vi "SubVI_Overlay Line(Offset) #.vi"(5 "ROI Descriptor":T2 {"Contours"."Type" items=["No Selection", "Point", "Line", "Rectangle", "Oval", "Polygon", "Freehand Region", "Annulus", "Unused2", "Unused3", "Broken Line", "Freehand Line", "Rotated Rectangle"]}, 7 "Perpendicular Line":T1, 9 "Fit Line":T1) -> (6 "Perpendicular Line(Offset)":T1, 8 "Fit Line(Offset)":T1)   [LabVIEW 2013]
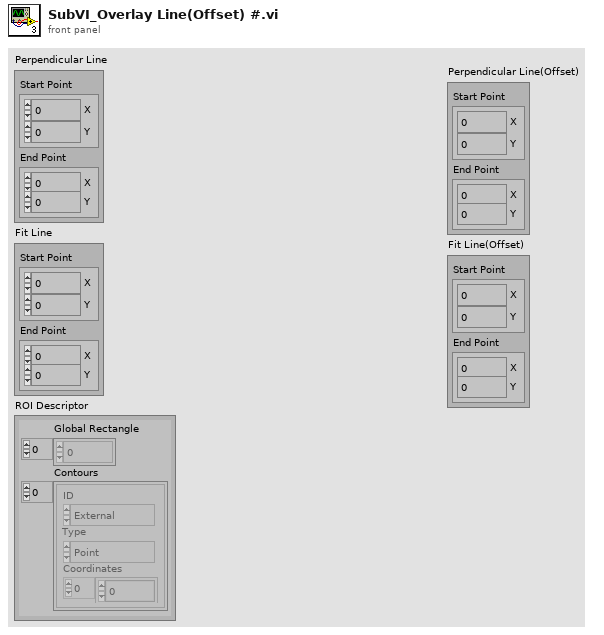
[diagram p1: front panel]
types:
  T1 = cluster{"Start Point":cluster{"X":i32, "Y":i32}, "End Point":cluster{"X":i32, "Y":i32}}
  T2 = typedef "ROI Descriptor" = cluster{"Global Rectangle":i32[], "Contours":cluster{"ID":enum32{"External", "Internal"}, "Type":u32, "Coordinates":i32[]}[]}
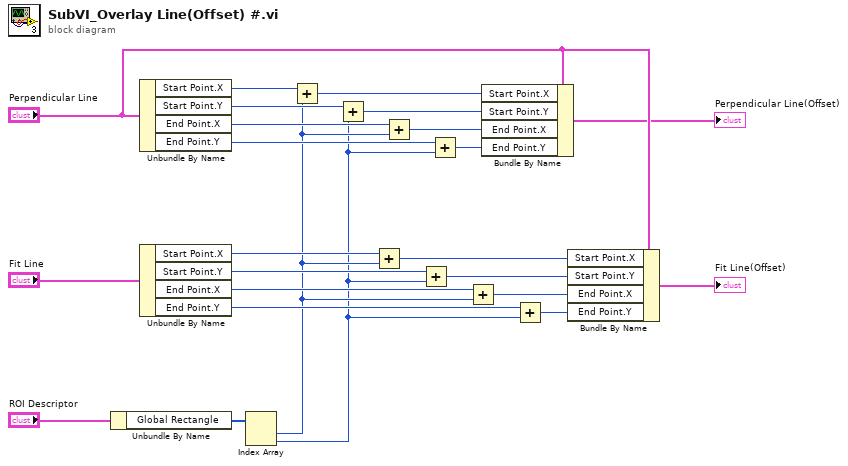
[diagram p0: block diagram]
diagram:
  n1 = Unbundle By Name("ROI Descriptor") -> ("Global Rectangle"=w22:i32[])
  n2 = Unbundle By Name("Perpendicular Line") -> ("Start Point.X"=w21:i32, "Start Point.Y"=w19:i32, "End Point.X"=w12:i32, "End Point.Y"=w11:i32)
  n3 = Unbundle By Name("Fit Line") -> ("Start Point.X"=w20:i32, "Start Point.Y"=w18:i32, "End Point.X"=w8:i32, "End Point.Y"=w7:i32)
  n4 = Index Array(array=w22) -> (element #1=w6:i32, element #2=w5:i32)  [unwired: 2 in]
  n5 = Add(x=w21, y=w6) -> (x+y=w17:i32)
  n6 = Add(x=w19, y=w5) -> (x+y=w16:i32)
  n7 = Add(x=w20, y=w6) -> (x+y=w14:i32)
  n8 = Add(x=w12, y=w6) -> (x+y=w9:i32)
  n9 = Add(x=w18, y=w5) -> (x+y=w13:i32)
  n10 = Add(x=w11, y=w5) -> (x+y=w10:i32)
  n11 = Add(x=w8, y=w6) -> (x+y=w4:i32)
  n12 = Bundle By Name(cluster="Perpendicular Line", "Start Point.X"=w17, "Start Point.Y"=w16, "End Point.X"=w9, "End Point.Y"=w10) -> (→"Perpendicular Line(Offset)":T1)
  n13 = Add(x=w7, y=w5) -> (x+y=w3:i32)
  n14 = Bundle By Name(cluster="Perpendicular Line", "Start Point.X"=w14, "Start Point.Y"=w13, "End Point.X"=w4, "End Point.Y"=w3) -> (→"Fit Line(Offset)":T1)
